vi "Start Acquiring.vi"(6 "wait for reply (T)":bool=TRUE, 8 "error in (no error)":errorcluster) -> (0 "error out":errorcluster, 1 "timed out?":bool, 2 "Reply Payload":T1)   [LabVIEW 2016, in "Impedance Data Acquisition and Decoding.lvlib"]
doc: "_____\nCreated using Delacor QMH Event Scripter 5.0.0.112."
uses:
  Impedance Data Acquisition and Decoding.lvlib
  Start Acquiring (Reply Payload)--cluster.ctl
  Start Acquiring Argument--cluster.ctl
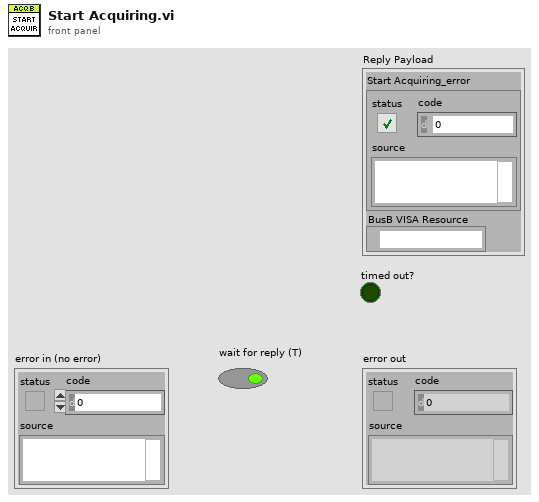
[diagram p1: front panel]
types:
  T1 = typedef "Impedance Data Acquisition and Decoding.lvlib/Start Acquiring (Reply Payload)--cluster.ctl" = cluster{"Start Acquiring_error":errorcluster, "BusB VISA Resource":refnum<visa-resource-name>}
  T2 = typedef "Impedance Data Acquisition and Decoding.lvlib/Request Events--cluster.ctl" = cluster{"Stop Module":refnum<user-event>, "Show Panel":refnum<user-event>, "Hide Panel":refnum<user-event>, "Get Module Execution Status":refnum<user-event>, "Show Diagram":refnum<user-event>, "Stop Acquiring":refnum<user-event>, "Change Settings":refnum<user-event>, "Start Acquiring":refnum<user-event>, "WakeUp Helper Loop":refnum<user-event>, "Initialize FINS":refnum<user-event>, "Initialize FINS for FTR":refnum<user-event>, "Initialize FINS for Qualification":refnum<user-event>}
  T3 = typedef "Impedance Data Acquisition and Decoding.lvlib/Start Acquiring Argument--cluster.ctl" = cluster{"Wait Notifier":refnum<notifier>, "wait for reply":bool}
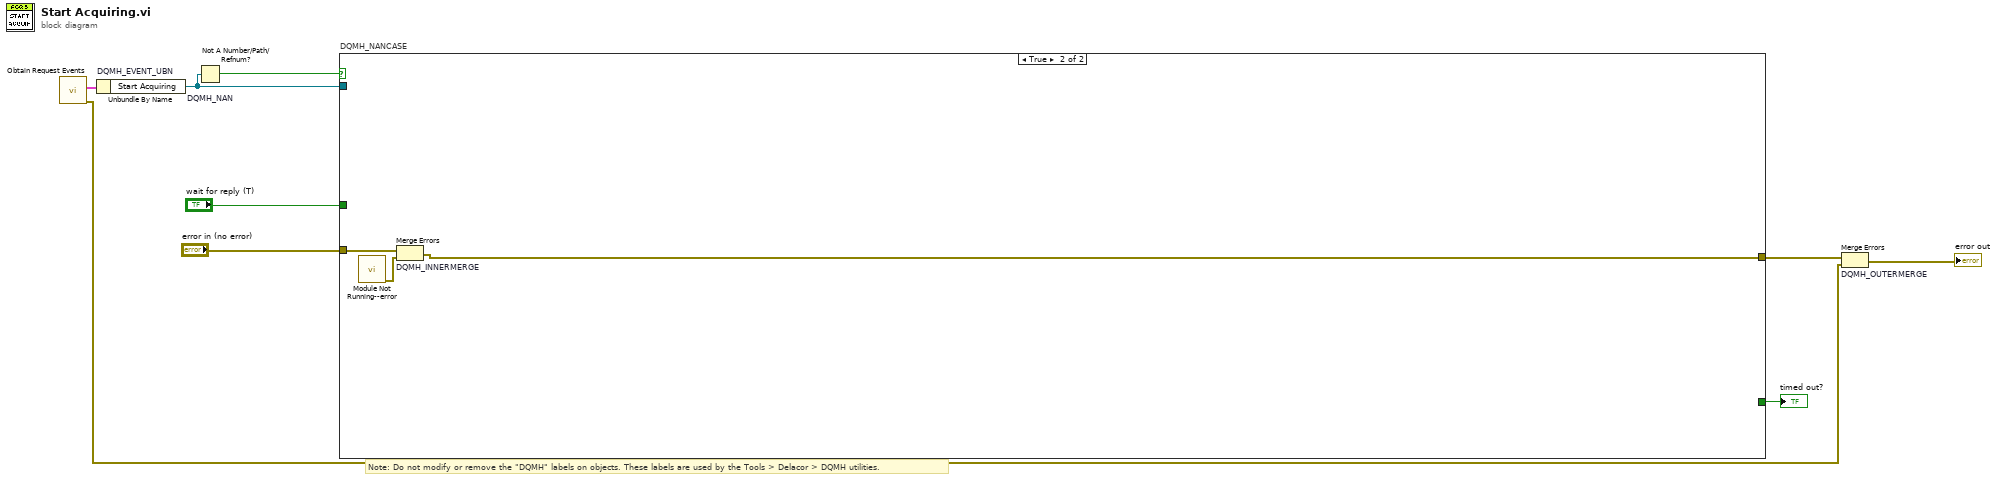
[diagram p0: block diagram]
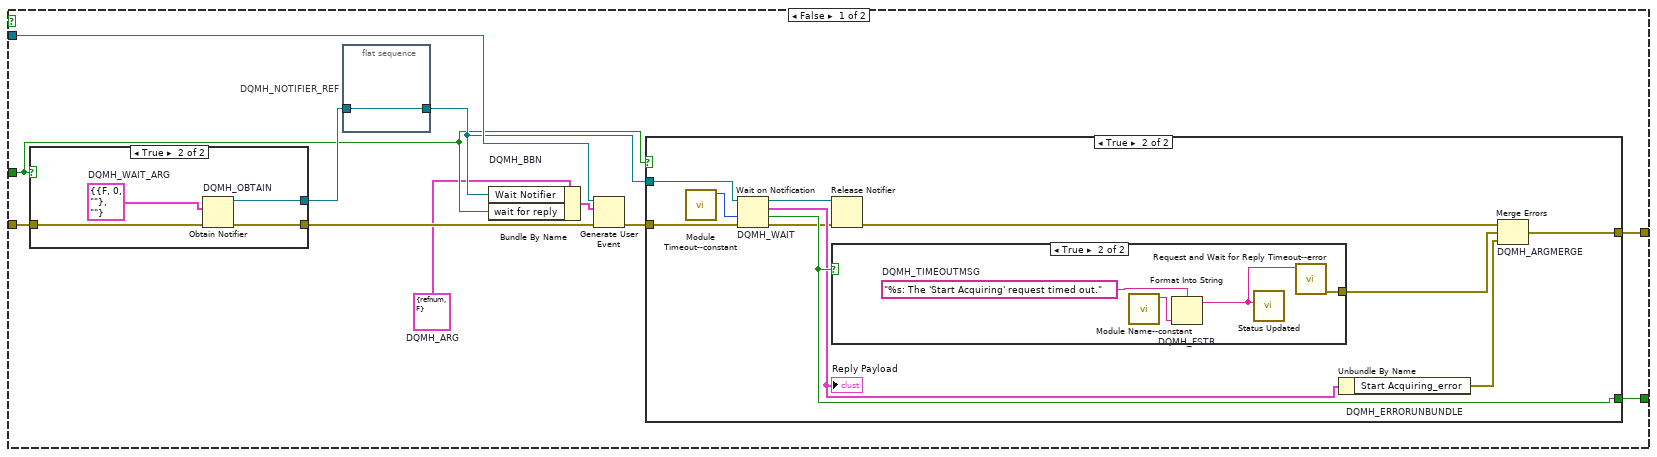
[diagram p2: hidden frame]
diagram:
  # "Note: Do not modify or remove the \"DQMH\" labels on objects. These labels are used by the Tools > Delacor > DQMH utilities."
  n1 = call "Obtain Request Events.vi"() -> ("error out"=w2:errorcluster, "FINS3-E BusB Data Acquisition and Decoding Request Events"=w1:T2)  [unwired: 10 in]
  n2 = Unbundle By Name "DQMH_EVENT_UBN"(w1) -> ("Start Acquiring"=w7:refnum<user-event>)
  n3 = Not A Number/Path/Refnum? "DQMH_NAN"(number/path/refnum=w7) -> (NaN/Path/Refnum?=w6:bool)
  n4 = case "DQMH_NANCASE" shown="True" w6 {
    tunnel: "error in (no error)" -> [w20 w45]
    tunnel: w7 -> [w18 _]
    tunnel: [w15 w44] -> w4
    tunnel: [w16 _] -> w5
    tunnel: "wait for reply (T)" -> [w11 _]
    frame False {
      w10 = T3 {"Wait Notifier"=refnum, "wait for reply"=FALSE}  # DQMH_ARG
      n5 = case shown="True" w11 {
        tunnel: w20 -> [w38 w42]
        tunnel: [w38 w41] -> w17
        tunnel: [_ w39] -> w13
        frame False {
        }
        frame True {
          w40 = T1 {"Start Acquiring_error"={"status"=FALSE, "code"=0, "source"=""}, "BusB VISA Resource"=""}  # DQMH_WAIT_ARG
          n6 = Obtain Notifier "DQMH_OBTAIN"(notification data type=w40, error in (no error)=w42) -> (notifier out=w39:refnum<notifier>, error out=w41:errorcluster)  [unwired: 2 in, 1 out]
        }
      }
      n7 = flat-sequence "DQMH_NOTIFIER_REF" {
        tunnel: w13 -> [w21]
        tunnel: [w21] -> w12
        frame #0 {
        }
      }
      n8 = Bundle By Name "DQMH_BBN"(cluster=w10, "Wait Notifier"=w12, "wait for reply"=w11) -> (w14:T3)
      n9 = Generate User Event(user event=w18, event data cluster=w14, error in=w17) -> (error out=w19:errorcluster)  [unwired: 1 in, 1 out]
      n10 = case shown="True" w11 {
        tunnel: w19 -> [w22 w33]
        tunnel: w12 -> [_ w32]
        tunnel: [_ w30] -> w16
        tunnel: [w22 w29] -> w15
        frame False {
        }
        frame True {
          n11 = call "Module Timeout--constant.vi"() -> ("Module Timeout"=w23:i32)  [unwired: 11 in]
          n12 = Wait on Notification "DQMH_WAIT"(notifier=w32, timeout in ms (-1)=w23, error in (no error)=w33) -> (notifier out=w31:refnum<notifier>, notification=w28:T1, timed out?=w30:bool, error out=w27:errorcluster)  [unwired: 1 in]
          "Reply Payload" <- w28
          n13 = Release Notifier(notifier=w31, error in (no error)=w27) -> (error out=w26:errorcluster)  [unwired: 1 in, 2 out]
          n14 = case shown="True" w30 {
            tunnel: [_ w35] -> w24
            frame False {
            }
            frame True {
              w37 = "%s: The 'Start Acquiring' request timed out."  # DQMH_TIMEOUTMSG
              n15 = call "Module Name--constant.vi"() -> ("Module Name"=w34:string)  [unwired: 11 in]
              n16 = Format Into String "DQMH_FSTR"(format string=w37, w34) -> (resulting string=w36:string)  [unwired: 2 in, 1 out]
              n17 = call "Status Updated.vi"("Status"=w36) -> ()  [unwired: 10 in, 1 out]
              n18 = call "Request and Wait for Reply Timeout--error.vi"("Error Message"=w36) -> ("error out"=w35:errorcluster)  [unwired: 10 in]
            }
          }
          n19 = Unbundle By Name "DQMH_ERRORUNBUNDLE"(w28) -> ("Start Acquiring_error"=w25:errorcluster)
          n20 = Merge Errors "DQMH_ARGMERGE"(w26, w24, w25) -> (w29:errorcluster)
        }
      }
    }
    frame True {
      n21 = call "Module Not Running--error.vi"() -> ("error out"=w43:errorcluster)  [unwired: 11 in]
      n22 = Merge Errors "DQMH_INNERMERGE"(w45, w43) -> (w44:errorcluster)
    }
  }
  "timed out?" <- w5
  n23 = Merge Errors "DQMH_OUTERMERGE"(w4, w2) -> (→"error out":errorcluster)
